vi "LV_2_DSC.vi"(8 "error in (no error)":errorcluster, 10 "data":T1[](array[typedef])) -> (0 "error out":errorcluster)   [LabVIEW 2016, in "VCL_2_DSC.lvclass"]
uses:
  VCL_2_DSC.lvclass
  typedefs/TSLtoLV-cluster.ctl
  <vilib>/lvdsc/historical/Open Trace (Numeric).vi
  <vilib>/lvdsc/historical/Write Trace (Numeric).vi
  <vilib>/lvdsc/NI_DSC.lvlib
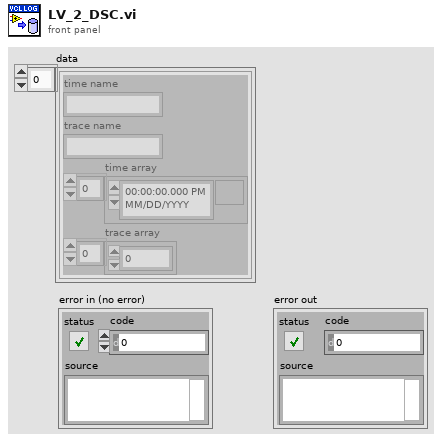
[diagram p1: front panel]
types:
  T1 = typedef "VCL_2_DSC.lvclass/TSLtoLV-cluster.ctl" = cluster{"time name":string, "trace name":string, "time array":timestamp[], "trace array":dbl[]}
  T2 = cluster{"show status bar (T)":bool, "compact (T)":bool, "use * as wildcard (F)":bool}
  T3 = cluster{"show status bar (T)":bool, "compact (T)":bool, "use * as wildcard (F)":bool, "delete data from source database (F)":bool}
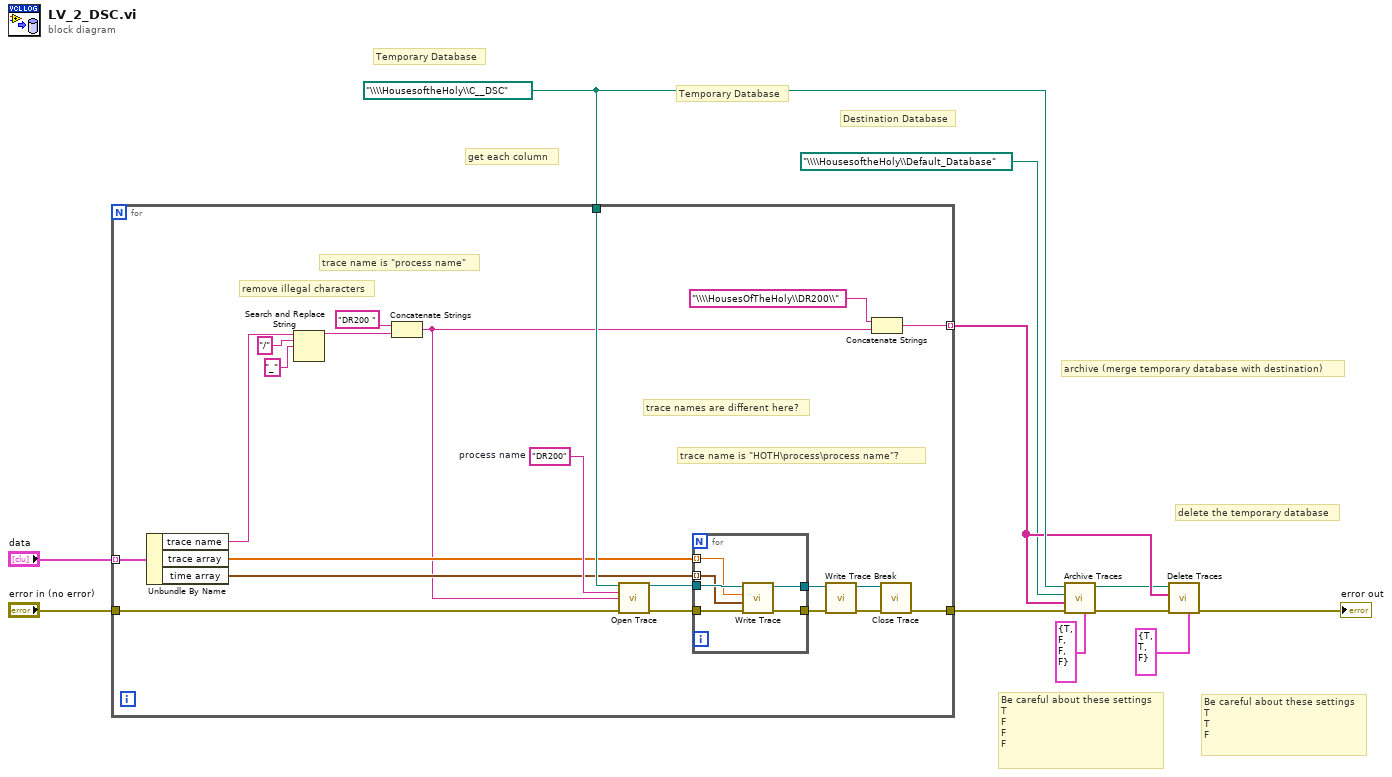
[diagram p0: block diagram]
diagram:
  w11 = path "\\\\HousesoftheHoly\\C__DSC" ("database URL")
  # "delete the temporary database"
  # "archive (merge temporary database with destination)"
  # "Temporary Database"
  # "Be careful about these settings\nT\nT\nF"
  # "Be careful about these settings\nT\nF\nF\nF"
  # "Temporary Database"
  # "Destination Database"
  # "get each column"
  n1 = for {
    tunnel: "data" -> [w20] mode=indexing
    tunnel: [w31] -> w8 mode=indexing
    tunnel: "error in (no error)" -> [w28]
    tunnel: [w27] -> w2
    tunnel: w11 -> [w22]
    w24 = "DR200"  # process name
    # "trace name is \"HOTH\\process\\process name\"?"
    # "trace name is \"process name\""
    # "remove illegal characters"
    # "trace names are different here?"
    n2 = Unbundle By Name(w20) -> ("trace name"=w19:string, "trace array"=w14:dbl[], "time array"=w13:timestamp[])
    n3 = Search and Replace String(input string=w19, search string="/", replace string="_" ("replace string (\"\")")) -> (result string=w29:string)  [unwired: 5 in, 3 out]
    n4 = Concatenate Strings("DR200 " ("process name"), w29) -> (w12:string)
    n5 = call-poly <vilib>:"Open Trace.vi"("database URL"=w22, "process name"=w24, "trace name"=w12, "error in (no error)"=w28) -> ("trace reference"=w25:refnum<k1>, "error out"=w26:errorcluster)  [unwired: 9 in, 1 out]
    n6 = for {
      tunnel: [w38] -> w18
      tunnel: [w37] -> w17
      tunnel: w25 -> [w36]
      tunnel: w26 -> [w35]
      tunnel: w13 -> [w34] mode=indexing
      tunnel: w14 -> [w33] mode=indexing
      n7 = call-poly <vilib>:"Write Trace.vi"("error in (no error)"=w35, "timestamp (now)"=w34, "value"=w33, "trace ref"=w36) -> ("error out"=w38:errorcluster, "trace ref out"=w37:refnum<k1>)  [unwired: 6 in]
    }
    n8 = call <vilib>:"Write Trace Break.vi"("error in (no error)"=w18, "trace ref"=w17) -> ("error out"=w16:errorcluster, "trace ref out"=w15:refnum<k1>)  [unwired: 8 in]
    n9 = Concatenate Strings("\\\\HousesOfTheHoly\\DR200\\" ("string"), w12) -> (w31:string)
    n10 = call <vilib>:"Close Trace.vi"("error in (no error)"=w16, "trace reference"=w15) -> ("error out"=w27:errorcluster)  [unwired: 9 in]
  }
  n11 = call <vilib>:"Archive Traces.vi"("options"=T3 {"show status bar (T)"=TRUE, "compact (T)"=FALSE, "use * as wildcard (F)"=FALSE, "delete data from source database (F)"=FALSE}, "error in (no error)"=w2, "trace names"=w8, "destination database URL"=path "\\\\HousesoftheHoly\\Default_Database", "source database URL"=w11) -> ("error out"=w9:errorcluster, "source database URL out"=w5:path)  [unwired: 4 in, 1 out]
  n12 = call <vilib>:"Delete Traces.vi"("options"=T2 {"show status bar (T)"=TRUE, "compact (T)"=TRUE, "use * as wildcard (F)"=FALSE}, "error in (no error)"=w9, "trace names"=w8, "database name"=w5) -> ("error out"=→"error out":errorcluster)  [unwired: 6 in, 1 out]
